vi "Select Worksheet.vi"   [LabVIEW 2026, in "XCel Report Engine.lvlib"]
uses:
  XCel Report Engine.lvlib
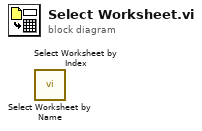
[diagram p0: block diagram]
diagram:
  n1 = call "Select Worksheet by Name.vi"() -> ()  [unwired: 3 in, 2 out]
  n2 = call "Select Worksheet by Index.vi"() -> ()  [unwired: 3 in, 2 out]
